vi "Joystick_Control_Testing_r1.vi"() -> ()   [LabVIEW 2015]
uses:
  <vilib>/Utility/inputDevices.llb/joystickAcquire.vi
  <vilib>/Utility/inputDevices.llb/closeJoystick.vi
panel:
  in  "unjam":bool
  out "Orientation complete":bool
  out "Winch going down":bool
  out "Full":bool
  out "Reverse Diff":dbl
  out "Forward Diff":dbl
  out "Scoop Position":dbl=0.9838866180000001
  out "Drum Accel x":dbl
  out "Winch Accel x":dbl
  in  "Scoops":dbl(knob)=0.075 min=0.05 max=0.1 step=0.005 scale=0.05..0.1
  in  "Winch":dbl(knob)=0.075 min=0.05 max=0.1 step=0.005 scale=0.05..0.1
  in  "Drum":dbl(knob)=0.075 min=0.05 max=0.1 step=0.005 scale=0.05..0.1
  in  "Disable Winch Auto Level":bool
  in  "Disable Drum Auto Level":bool
  out "Current Template - Right":T1(ring)=enum."Range 2"
  out "Current Template - Left":T1(ring)=enum."Range 2"
  in  "Dead wheel speed":dbl(slide)=0.03 min=0.0 max=0.1666 step=0.01 scale=0.0..0.1666
  in  "Stop":bool
  in  "Manual control":bool
  in  "Dump or Mine":dbl(knob) min=-1.0 max=1.0 step=1.0 scale=-1.0..1.0
  in  "stop 2":bool
  out "loc_theta":dbl
  out "loc_y":dbl
  out "loc_x":dbl
  out "Position_Lock":bool
  out "RIGHT_BEACON_BOOL_array":bool[](array[boolean])
  out "LEFT_BEACON_BOOL_array":bool[](array[boolean])
  in  "Start Run":bool
  in  "Auto/Manual":bool
  out "Reverse DC":dbl=0.5
  out "Forward DC":dbl=0.5
  out "Ratio Forward":dbl
  out "Reverse":bool
  out "Right Duty Cycle":dbl=0.5
  out "Left Duty Cycle":dbl=0.5
  out "Right Turn":bool
  out "Left Turn":bool
  in  "stop":bool
  out "Y axis":i32
  out "X axis":i32
  # "1 is the dumping position"
  # "Auto = true\nMaunal = false"
  # "zero is level"
  # "Reverse"
  # "Forward"
  # "Up"
  # "Down"
  # "CW"
  # "CCW"
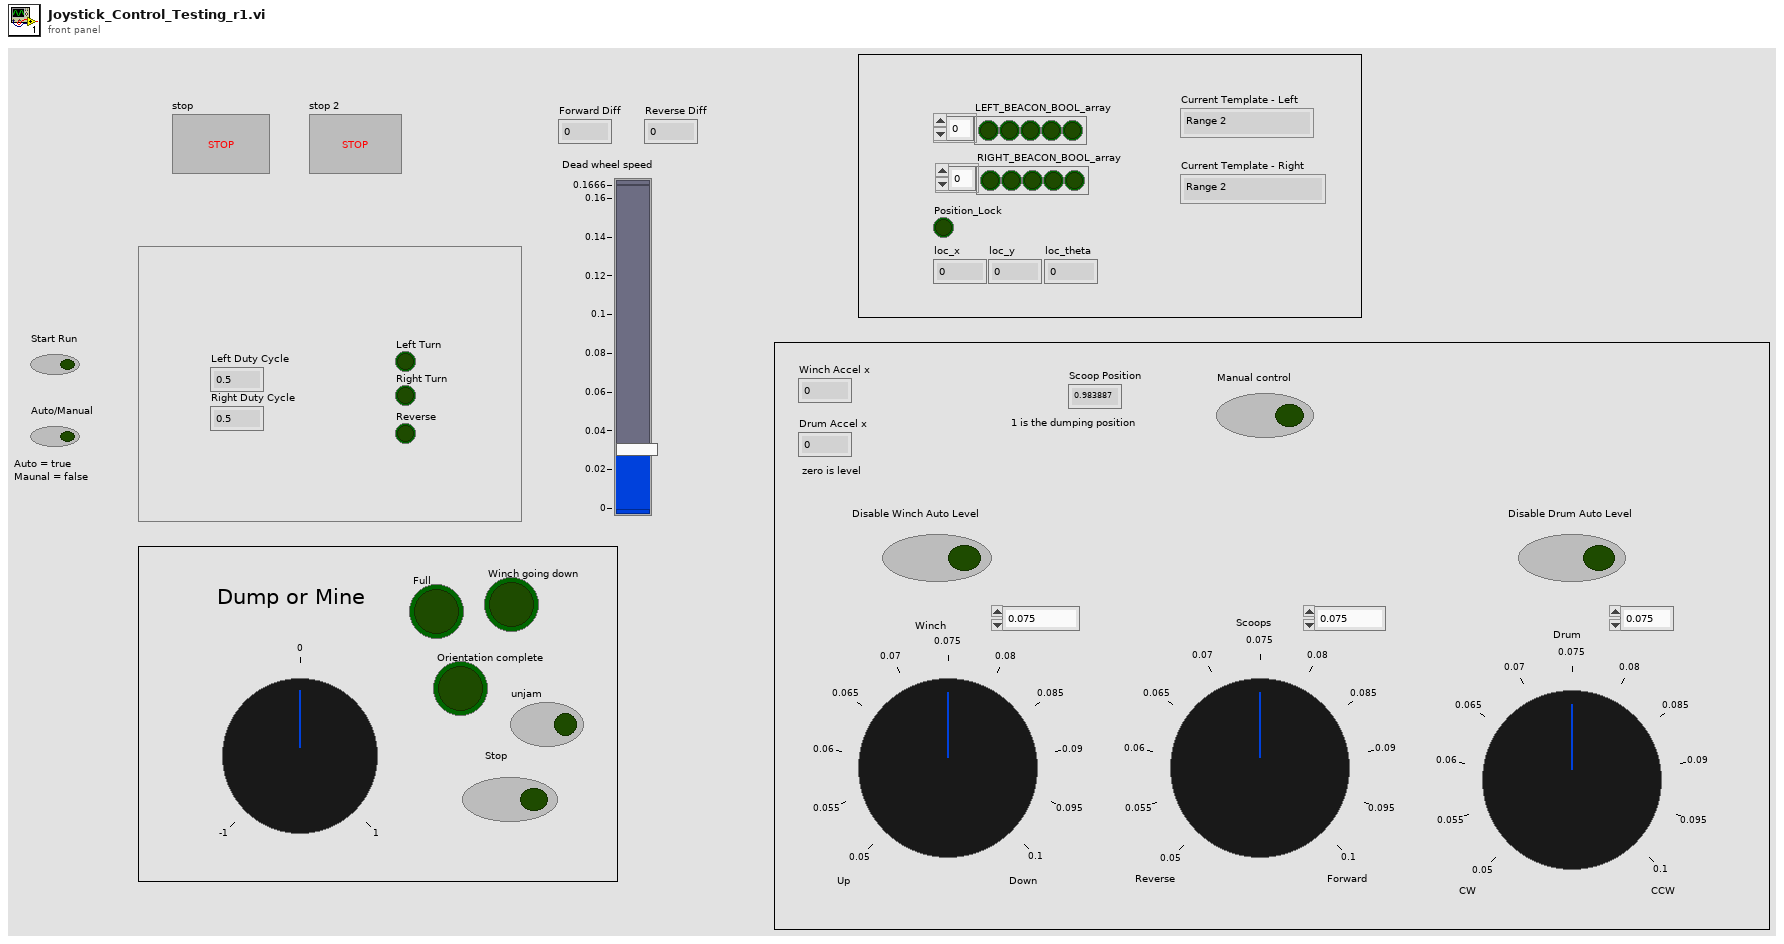
[diagram p1: front panel]
types:
  T1 = enum16{"Range 1", "Range 2", "Range 3", "Range 0"}
  T2 = cluster{"Lock":bool, "Current Valid":bool, "Current Template":enum16{"Range 1", "Range 2", "Range 3", "Range 0"}, "Tracking Coordinates":cluster{"X":dbl, "Y":dbl}, "Setting Values":cluster{"Min Score":dbl, "Min Scale":dbl, "Max Scale":dbl, "Curve Parameters":cluster{"Min Length":i32, "Row Search Step":i32, "Col Search Step":i32}}}
  T3 = cluster{"X axis":i32, "Y axis":i32, "Z axis":i32, "X axis rotation":i32, "Y axis rotation":i32, "Z axis rotation":i32, "U axis":i32, "V axis":i32}
  T4 = cluster{"button 1":bool, "button 2":bool, "button 3":bool, "button 4":bool, "button 5":bool, "button 6":bool, "button 7":bool, "button 8":bool, "button 9":bool, "button 10":bool, "button 11":bool, "button 12":bool, "button 13":bool, "button 14":bool, "button 15":bool, "button 16":bool, "button 17":bool, "button 18":bool, "button 19":bool, "button 20":bool, "button 21":bool, "button 22":bool, "button 23":bool, "button 24":bool, "button 25":bool, "button 26":bool, "button 27":bool, "button 28":bool, "button 29":bool, "button 30":bool, "button 31":bool, "button 32":bool}
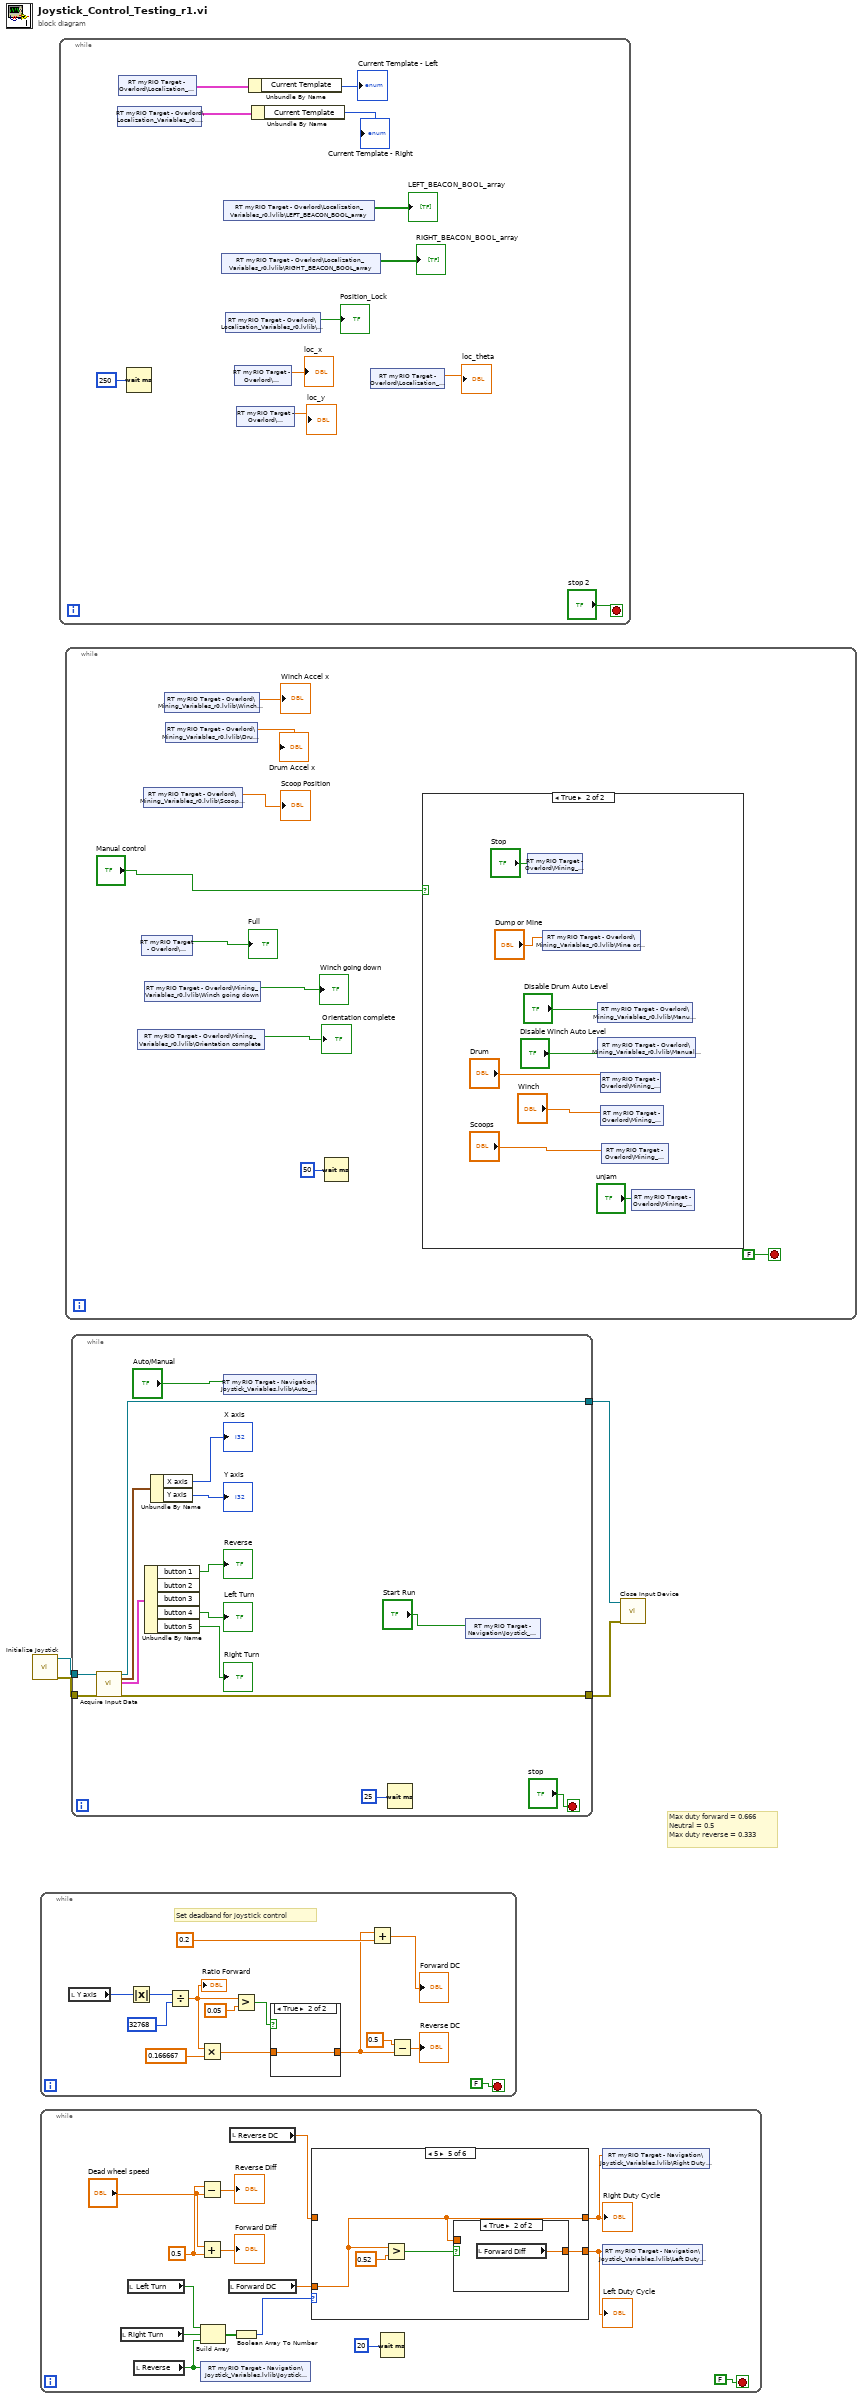
[diagram p0: block diagram]
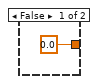
[diagram p3: hidden frame]
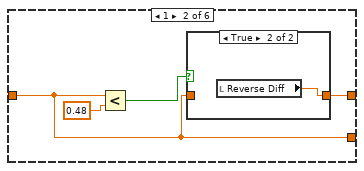
[diagram p5: hidden frame]
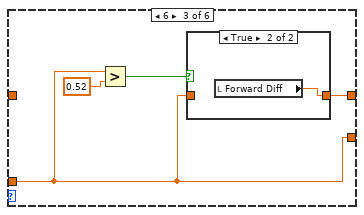
[diagram p7: hidden frame]
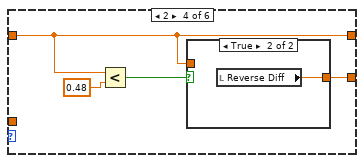
[diagram p9: hidden frame]
diagram:
  # "Max duty forward = 0.666\nNeutral = 0.5\nMax duty reverse = 0.333"
  n1 = call <vilib>:"Initialize Joystick.vi"() -> ("error out"=w2:errorcluster, "device ID"=w4:refnum<k1>)  [unwired: 10 in]
  n2 = while {
    stop <- FALSE stop-if-true
    # "Set deadband for joystick control"
    n3 = local read "Y axis"() -> (w18:i32)
    n4 = Absolute Value(x=w18) -> (abs(x)=w17:i32)
    n5 = Divide(x=w17, y=32768) -> (x/y=w5:dbl)
    "Ratio Forward" <- w5
    n6 = Multiply(x=w5, y=0.166667) -> (x*y=w8:dbl)
    n7 = Greater?(x=w5, y=0.05) -> (0:w6:bool)
    n8 = case shown="True" w6 {
      tunnel: [0.0 ("y") w20] -> w9
      tunnel: w8 -> [_ w20]
      frame False {
      }
      frame True {
      }
    }
    n9 = Add(x=w9, y=0.2) -> (x+y=→"Forward DC":dbl)
    n10 = Subtract(x=0.5, y=w9) -> (x-y=→"Reverse DC":dbl)
  }
  n11 = while {
    stop <- FALSE stop-if-true
    w22 = 0.5
    n12 = local read "Right Turn"() -> (w33:bool)
    n13 = local read "Left Turn"() -> (w34:bool)
    n14 = local read "Reverse"() -> (w25:bool)
    n15 = Subtract(x=w22, y="Dead wheel speed") -> (x-y=→"Reverse Diff":dbl)
    n16 = Add(x="Dead wheel speed", y=w22) -> (x+y=→"Forward Diff":dbl)
    n17 = Build Array(w34, w33, w25) -> (w32:bool[])
    n18 = shared-variable "RT myRIO Target - Navigation\\Joystick_Variables.lvlib\\Joystick Direction"(w25) -> ()  [unwired: 1 in, 1 out]
    n19 = local read "Forward DC"() -> (w28:dbl)
    n20 = local read "Reverse DC"() -> (w27:dbl)
    n21 = Boolean Array To Number(Boolean array=w32) -> (number=w35:u32)
    n22 = case shown="5" w35 {
      tunnel: [w36 w37 w43 w50 w56 w61] -> w29
      tunnel: [w36 w38 w44 w49 w55 w61] -> w30
      tunnel: w28 -> [_ _ w43 _ w55 w61]
      tunnel: w27 -> [w36 w37 _ w49 _ _]
      frame 0, Default {
      }
      frame 1 {
        n23 = Less?(x=w37, y=0.48) -> (x < y?=w40:bool)
        n24 = case shown="True" w40 {
          tunnel: [w41 w42] -> w38
          tunnel: w37 -> [w41 _]
          frame False {
          }
          frame True {
            n25 = local read "Reverse Diff"() -> (w42:dbl)
          }
        }
      }
      frame 6 {
        n26 = Greater?(x=w43, y=0.52) -> (0:w46:bool)
        n27 = case shown="True" w46 {
          tunnel: [w47 w48] -> w44
          tunnel: w43 -> [w47 _]
          frame False {
          }
          frame True {
            n28 = local read "Forward Diff"() -> (w48:dbl)
          }
        }
      }
      frame 2 {
        n29 = Less?(x=w49, y=0.48) -> (x < y?=w51:bool)
        n30 = case shown="True" w51 {
          tunnel: [w53 w54] -> w50
          tunnel: w49 -> [w53 _]
          frame False {
          }
          frame True {
            n31 = local read "Reverse Diff"() -> (w54:dbl)
          }
        }
      }
      frame 5 {
        n32 = Greater?(x=w55, y=0.52) -> (0:w57:bool)
        n33 = case shown="True" w57 {
          tunnel: [w59 w60] -> w56
          tunnel: w55 -> [w59 _]
          frame False {
          }
          frame True {
            n34 = local read "Forward Diff"() -> (w60:dbl)
          }
        }
      }
      frame 4 {
      }
    }
    "Left Duty Cycle" <- w29
    "Right Duty Cycle" <- w30
    n35 = Wait (ms)(milliseconds to wait=u32 20) -> ()  [unwired: 1 out]
    n36 = shared-variable "RT myRIO Target - Navigation\\Joystick_Variables.lvlib\\Right Duty Cycle"(w30) -> ()  [unwired: 1 in, 1 out]
    n37 = shared-variable "RT myRIO Target - Navigation\\Joystick_Variables.lvlib\\Left Duty Cycle"(w29) -> ()  [unwired: 1 in, 1 out]
  }
  n38 = while {
    stop <- "stop 2" stop-if-true
    n39 = shared-variable "RT myRIO Target - Overlord\\Localization_Variables_r0.lvlib\\Info - Right"() -> (w64:T2)  [unwired: 1 in, 1 out]
    n40 = shared-variable "RT myRIO Target - Overlord\\Localization_Variables_r0.lvlib\\Info - Left"() -> (w65:T2)  [unwired: 1 in, 1 out]
    n41 = Wait (ms)(milliseconds to wait=u32 250) -> ()  [unwired: 1 out]
    n42 = shared-variable "RT myRIO Target - Overlord\\Localization_Variables_r0.lvlib\\RIGHT_BEACON_BOOL_array"() -> (→"RIGHT_BEACON_BOOL_array":bool[])  [unwired: 1 in, 1 out]
    n43 = shared-variable "RT myRIO Target - Overlord\\Localization_Variables_r0.lvlib\\LEFT_BEACON_BOOL_array"() -> (→"LEFT_BEACON_BOOL_array":bool[])  [unwired: 1 in, 1 out]
    n44 = shared-variable "RT myRIO Target - Overlord\\Localization_Variables_r0.lvlib\\Position_Lock"() -> (→"Position_Lock":bool)  [unwired: 1 in, 1 out]
    n45 = shared-variable "RT myRIO Target - Overlord\\Localization_Variables_r0.lvlib\\loc_x"() -> (→"loc_x":dbl)  [unwired: 1 in, 1 out]
    n46 = shared-variable "RT myRIO Target - Overlord\\Localization_Variables_r0.lvlib\\loc_y"() -> (→"loc_y":dbl)  [unwired: 1 in, 1 out]
    n47 = Unbundle By Name(w65) -> ("Current Template"=→"Current Template - Left":T1)
    n48 = Unbundle By Name(w64) -> ("Current Template"=→"Current Template - Right":T1)
    n49 = shared-variable "RT myRIO Target - Overlord\\Localization_Variables_r0.lvlib\\loc_theta"() -> (→"loc_theta":dbl)  [unwired: 1 in, 1 out]
  }
  n50 = while {
    stop <- FALSE stop-if-true
    n51 = shared-variable "RT myRIO Target - Overlord\\Mining_Variables_r0.lvlib\\Orientation complete"() -> (→"Orientation complete":bool)  [unwired: 1 in, 1 out]
    n52 = shared-variable "RT myRIO Target - Overlord\\Mining_Variables_r0.lvlib\\Full"() -> (→"Full":bool)  [unwired: 1 in, 1 out]
    n53 = shared-variable "RT myRIO Target - Overlord\\Mining_Variables_r0.lvlib\\Scoop Position"() -> (→"Scoop Position":dbl)  [unwired: 1 in, 1 out]
    n54 = shared-variable "RT myRIO Target - Overlord\\Mining_Variables_r0.lvlib\\Winch going down"() -> (→"Winch going down":bool)  [unwired: 1 in, 1 out]
    n55 = shared-variable "RT myRIO Target - Overlord\\Mining_Variables_r0.lvlib\\Winch Accel x"() -> (→"Winch Accel x":dbl)  [unwired: 1 in, 1 out]
    n56 = shared-variable "RT myRIO Target - Overlord\\Mining_Variables_r0.lvlib\\Drum Accel x"() -> (→"Drum Accel x":dbl)  [unwired: 1 in, 1 out]
    n57 = Wait (ms)(milliseconds to wait=u32 50) -> ()  [unwired: 1 out]
    n58 = case shown="True" "Manual control" {
      frame False {
      }
      frame True {
        n59 = shared-variable "RT myRIO Target - Overlord\\Mining_Variables_r0.lvlib\\Stop"("Stop") -> ()  [unwired: 1 in, 1 out]
        n60 = shared-variable "RT myRIO Target - Overlord\\Mining_Variables_r0.lvlib\\Mine or Dump"("Dump or Mine") -> ()  [unwired: 1 in, 1 out]
        n61 = shared-variable "RT myRIO Target - Overlord\\Mining_Variables_r0.lvlib\\Manual Drum"("Disable Drum Auto Level") -> ()  [unwired: 1 in, 1 out]
        n62 = shared-variable "RT myRIO Target - Overlord\\Mining_Variables_r0.lvlib\\Manual Winch"("Disable Winch Auto Level") -> ()  [unwired: 1 in, 1 out]
        n63 = shared-variable "RT myRIO Target - Overlord\\Mining_Variables_r0.lvlib\\Drum"("Drum") -> ()  [unwired: 1 in, 1 out]
        n64 = shared-variable "RT myRIO Target - Overlord\\Mining_Variables_r0.lvlib\\Winch"("Winch") -> ()  [unwired: 1 in, 1 out]
        n65 = shared-variable "RT myRIO Target - Overlord\\Mining_Variables_r0.lvlib\\Scoops"("Scoops") -> ()  [unwired: 1 in, 1 out]
        n66 = shared-variable "RT myRIO Target - Overlord\\Mining_Variables_r0.lvlib\\unjam"("unjam") -> ()  [unwired: 1 in, 1 out]
      }
    }
  }
  n67 = while {
    tunnel: w4 -> [w105]
    tunnel: [w104] -> w3
    tunnel: w2 -> [w103]
    tunnel: [w102] -> w1
    stop <- "stop" stop-if-true
    n68 = call-poly <vilib>:"Acquire Input Data.vi"("device ID"=w105, "error in (no error)"=w103) -> ("device ID"=w104:refnum<k1>, "axis info"=w101:T3, "button info"=w100:T4, "error out"=w102:errorcluster)  [unwired: 13 in, 1 out]
    n69 = Unbundle By Name(w100) -> ("button 1"=→"Reverse":bool, "button 4"=→"Left Turn":bool, "button 5"=→"Right Turn":bool)  [unwired: 2 out]
    n70 = Unbundle By Name(w101) -> ("X axis"=→"X axis":i32, "Y axis"=→"Y axis":i32)
    n71 = shared-variable "RT myRIO Target - Navigation\\Joystick_Variables.lvlib\\Auto_Manual"("Auto/Manual") -> ()  [unwired: 1 in, 1 out]
    n72 = Wait (ms)(milliseconds to wait=u32 25) -> ()  [unwired: 1 out]
    n73 = shared-variable "RT myRIO Target - Navigation\\Joystick_Variables.lvlib\\Start Run"("Start Run") -> ()  [unwired: 1 in, 1 out]
  }
  n74 = call-poly <vilib>:"Close Input Device.vi"("error in (no error)"=w1, "device ID"=w3) -> ()  [unwired: 8 in, 1 out]
